vi "Value to tri-colour map.vi"(1 "Vmax":sgl=1.0, 2 "Vmin":sgl=-1.0, 3 "V":sgl) -> (0 "Colour out":T1={"Red"=0.25, "Green"=0.5, "Blue"=0.25, "Alpha"=1.0})   [LabVIEW 2017]
uses:
  <vilib>/Utility/miscctls.llb/LVRGBAColorTypeDef.ctl
panel:
  # "Bernstein polynomials to generate RGB colour values"
  # "PN 23/10/17"
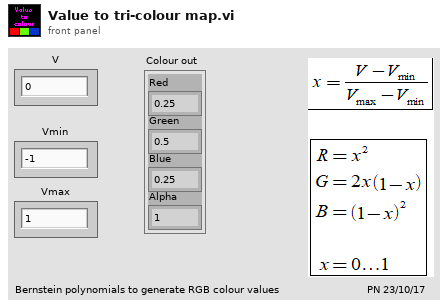
[diagram p1: front panel]
types:
  T1 = typedef "LVRGBAColorTypeDef.ctl" = cluster{"Red":sgl, "Green":sgl, "Blue":sgl, "Alpha":sgl}
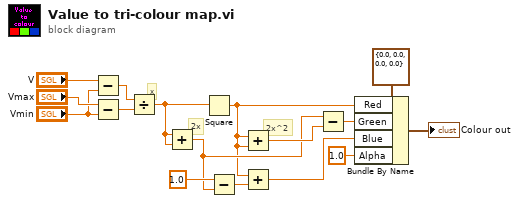
[diagram p0: block diagram]
diagram:
  # "2x^2"
  # "2x"
  # "x"
  n1 = Subtract(x="V", y="Vmin") -> (x-y=w13:sgl)
  n2 = Subtract(x="Vmax", y="Vmin") -> (x-y=w12:sgl)
  n3 = Divide(x=w13, y=w12) -> (x/y=w7:sgl)
  n4 = Add(x=w7, y=w7) -> (x+y=w4:sgl)
  n5 = Square(x=w7) -> (x^2=w2:sgl)
  n6 = Subtract(x=sgl 1.0, y=w4) -> (x-y=w3:sgl)
  n7 = Add(x=w2, y=w2) -> (x+y=w6:sgl)
  n8 = Add(x=w2, y=w3) -> (x+y=w1:sgl)
  n9 = Subtract(x=w4, y=w6) -> (x-y=w5:sgl)
  n10 = Bundle By Name(cluster=T1 {"Red"=0.0, "Green"=0.0, "Blue"=0.0, "Alpha"=0.0} ("RGBA Color"), "Red"=w2, "Green"=w5, "Blue"=w1, "Alpha"=sgl 1.0) -> (→"Colour out":T1)
